vi "getSensorInfo.vi"(8 "error in (no error)":errorcluster, 11 "Camera in":refnum<class "Camera.lvclass">) -> (0 "error out":errorcluster, 2 "PCO_SensorInfo":T1 {"iSensorInfoBits" format="%x"}, 3 "Camera out":refnum<class "Camera.lvclass">)   [LabVIEW 2019, in "Camera.lvclass"]
doc: "Get image sensor parameters required for setting up the convert controls"
uses:
  Camera.lvclass
  Camera.lvclass/Camera.ctl
  pco.convert/Convert.lvlib
  pco.sdk/ImageInformation/ImageInformation.lvlib
  pco.sdk/GeneralCameraStatus/GeneralCameraStatus.lvlib
  pco.sdk/ImageSensor/ImageSensor.lvlib
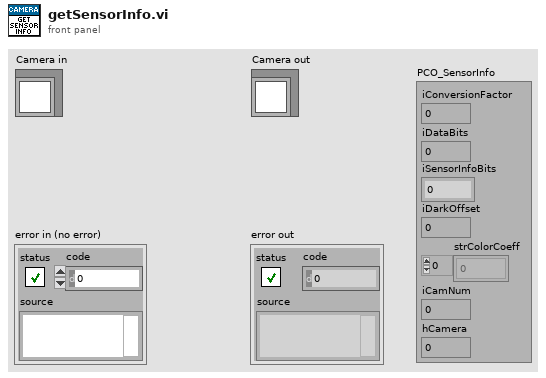
[diagram p1: front panel]
types:
  T1 = cluster{"iConversionFactor":i32, "iDataBits":i32, "iSensorInfoBits":i32, "iDarkOffset":i32, "strColorCoeff":dbl[], "iCamNum":i32, "hCamera":u64}
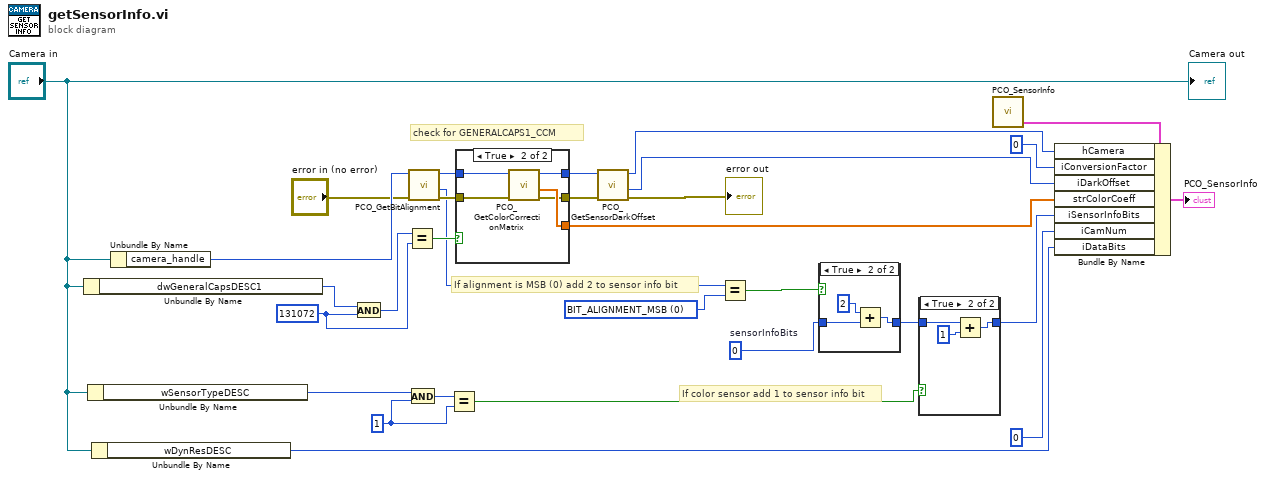
[diagram p0: block diagram]
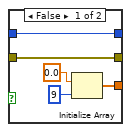
[diagram p4: hidden frame]
diagram:
  w2 = u16 0 items=["BIT_ALIGNMENT_MSB", "BIT_ALIGNMENT_LSB"] ("wBitAlignment")
  w18 = u16 1 ("y")
  w21 = 0  # sensorInfoBits
  w27 = u32 131072 ("y")
  # "If color sensor add 1 to sensor info bit"
  # "If alignment is MSB (0) add 2 to sensor info bit"
  # "check for GENERALCAPS1_CCM"
  n1 = Unbundle By Name("Camera in") -> ("dwGeneralCapsDESC1"=w28:u32)
  n2 = Unbundle By Name("Camera in") -> ("wSensorTypeDESC"=w20:u16)
  n3 = Unbundle By Name("Camera in") -> ("wDynResDESC"=w4:u16)
  n4 = Unbundle By Name("Camera in") -> ("camera_handle"=w30:u64)
  n5 = And(x=w28, y=w27) -> (x .and. y?=w1:u32)
  n6 = Equal?(x=w1, y=w27) -> (x = y?=w26:bool)
  n7 = And(x=w20, y=w18) -> (x .and. y?=w19:u16)
  n8 = call "PCO_GetBitAlignment.vi"("error in (no error)"="error in (no error)", "ph"=w30) -> ("error out"=w24:errorcluster, "wBitAlignment"=w23:u16, "ph out"=w25:u64)  [unwired: 6 in, 1 out]
  n9 = Equal?(x=w19, y=w18) -> (x = y?=w17:bool)
  n10 = case shown="True" w26 {
    tunnel: w25 -> [w31 w40]
    tunnel: w24 -> [w32 w39]
    tunnel: [w33 w38] -> w6
    tunnel: [w32 w37] -> w14
    tunnel: [w31 w36] -> w15
    frame False {
      n11 = Initialize Array(0.0 ("element"), 9 ("dimension size")) -> (w33:dbl[])
    }
    frame True {
      n12 = call "PCO_GetColorCorrectionMatrix.vi"("error in (no error)"=w39, "ph"=w40) -> ("error out"=w37:errorcluster, "pdMatrix"=w38:dbl[], "ph out"=w36:u64)  [unwired: 6 in, 1 out]
    }
  }
  n13 = call "PCO_GetSensorDarkOffset.vi"("error in (no error)"=w14, "ph"=w15) -> ("error out"=→"error out":errorcluster, "wDarkOffset"=w8:u16, "ph out"=w9:u64)  [unwired: 6 in, 1 out]
  n14 = Equal?(x=w23, y=w2) -> (x = y?=w22:bool)
  n15 = case shown="True" w22 {
    tunnel: w21 -> [w41 w44]
    tunnel: [w41 w42] -> w16
    frame False {
    }
    frame True {
      n16 = Add(x=2, y=w44) -> (x+y=w42:i32)
    }
  }
  n17 = case shown="True" w17 {
    tunnel: w16 -> [w45 w48]
    tunnel: [w45 w46] -> w7
    frame False {
    }
    frame True {
      n18 = Add(x=w48, y=1) -> (x+y=w46:i32)
    }
  }
  n19 = call "PCO_SensorInfo.vi"() -> ("PCO_SensorInfo"=w12:T1)  [unwired: 4 in, 4 out]
  n20 = Bundle By Name(cluster=w12, "hCamera"=w9, "iConversionFactor"=0, "iDarkOffset"=w8, "strColorCoeff"=w6, "iSensorInfoBits"=w7, "iCamNum"=0, "iDataBits"=w4) -> (→"PCO_SensorInfo":T1)
  "Camera out" <- "Camera in"
